vi "RemoveAllSubpanel.vi"(11 "SubRef":refnum<vi>[](array[refnum])) -> ()   [LabVIEW 2020, in "Other.lvlib"]
uses:
  Other.lvlib
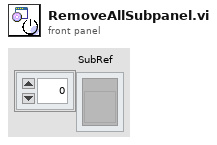
[diagram p1: front panel]
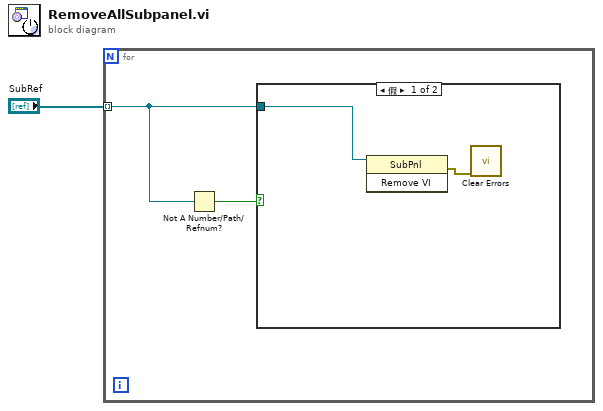
[diagram p0: block diagram]
diagram:
  n1 = for {
    tunnel: "SubRef" -> [w3] mode=indexing
    n2 = Not A Number/Path/Refnum?(number/path/refnum=w3) -> (NaN/Path/Refnum?=w2:bool)
    n3 = case shown="假" w2 {
      tunnel: w3 -> [w5 _]
      frame False {
        n4 = invoke class="SubPnl" method="Remove VI"(reference=w5) -> (error out=w4:errorcluster)  [unwired: 2 in, 2 out]
        n5 = call <vilib>:"Clear Errors.vi"("error in (no error)"=w4) -> ()  [unwired: 5 in, 2 out]
      }
      frame True {
      }
    }
  }
